vi "Read Sample.vi"(0 "TDMS In":refnum<k34>, 11 "Error In":errorcluster) -> (4 "TDMS Out":refnum<k34>, 6 "Input Vector":dbl[](array[numeric]), 8 "Output Vector":dbl[](array[numeric]), 14 "EOF?":bool, 15 "Error Out":errorcluster)   [LabVIEW 2015, in "Teaching File.lvlib"]
doc: "Read multiple teaching samples from TDMS file. Teaching_Data is the group read for the data. The TDMS channel ordering is used for the order of inputs and outputs.\n\nNumeric values in che channel name is not used for ordering the columns.\n\nIf end of file is reached, the Read_Index is set to 0, preparing for another read from the start of the file."
uses:
  Teaching File.lvlib
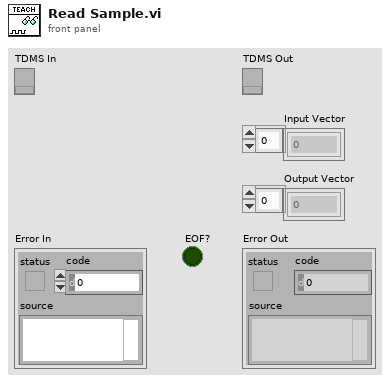
[diagram p1: front panel]
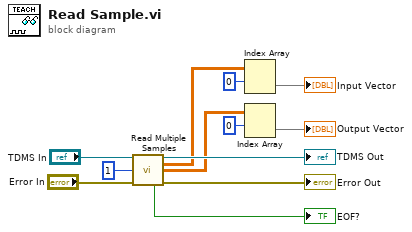
[diagram p0: block diagram]
diagram:
  n1 = call "Read Multiple Samples.vi"("TDMS In"="TDMS In", "#samples (-1: all)"=i64 1, "Error In"="Error In") -> ("TDMS Out"=→"TDMS Out":refnum<k34>, "Input Vectors"=w8:dbl[][], "Output Vectors"=w4:dbl[][], "EOF?"=→"EOF?":bool, "Error Out"=→"Error Out":errorcluster)  [unwired: 8 in]
  n2 = Index Array(array=w8, index (row)=0) -> (element=→"Input Vector":dbl[])  [unwired: 1 in]
  n3 = Index Array(array=w4, index (row)=0) -> (element=→"Output Vector":dbl[])  [unwired: 1 in]
